vi "Save Recall Instrument Settings.vi"(8 "error in (no error)":errorcluster, 9 "Memory Location (0)":u32 max=99 step=1 format="%#_0f", 10 "Save Recall Settings (0:Save)":u16(ring) items=["Save", "Recall"], 11 "VISA resource name":refnum<visa-resource-name>) -> (0 "error out":errorcluster, 3 "VISA resource name out":refnum<visa-resource-name>)   [LabVIEW 2015, in "BK Precision 983X Series.lvlib"]
doc: "Saves or recalls instrument settings to or from a specified memory location from internal memory or from a connected external USB flash memory."
uses:
  <instrlib>/BK Precision 983X Series/BK Precision 983X Series.lvlib
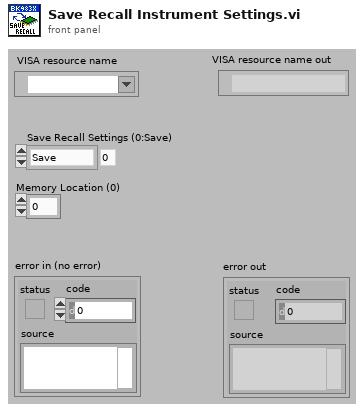
[diagram p1: front panel]
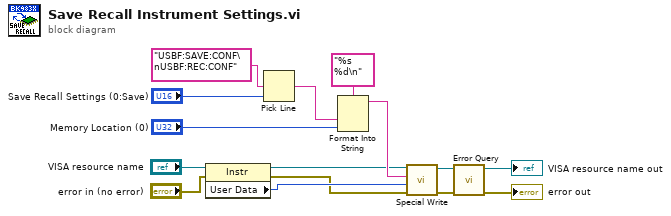
[diagram p0: block diagram]
diagram:
  n1 = property class="Instr"(reference="VISA resource name", error in="error in (no error)") -> (reference out=w1:refnum<visa-resource-name>, error out=w2:errorcluster, "User Data"=w3:u32)
  n2 = Pick Line(multi-line string="USBF:SAVE:CONF\nUSBF:REC:CONF", line index="Save Recall Settings (0:Save)") -> (output string=w11:string)  [unwired: 1 in]
  n3 = Format Into String(format string="%s %d\n", w11, "Memory Location (0)") -> (resulting string=w6:string)  [unwired: 2 in, 1 out]
  n4 = call <instrlib>:"Special Write.vi"("error in (no error)"=w2, "Delay (0 ms)"=w3, "Input String"=w6, "VISA resource name"=w1) -> ("error out"=w7:errorcluster, "VISA resource name out"=w8:refnum<visa-resource-name>)  [unwired: 6 in]
  n5 = call <instrlib>:"Error Query.vi"("error in (no error)"=w7, "VISA resource name"=w8) -> ("error out"=→"error out":errorcluster, "VISA resource name out"=→"VISA resource name out":refnum<visa-resource-name>)  [unwired: 6 in, 2 out]
